vi "NI 5783 - Getting Started (FPGA).vi"() -> ()   [LabVIEW 2017]
doc: "Example Description:\nThis example acquires records of analog input data and generates analog output data from the NI 5783 adapter module. For the analog input, it allows the user to select an AI channel, trigger type, and record size. For the analog output, it allows the user to select AO channel, waveform signal type, frequency, amplitude, and sampling information. This VI is compiled for all FPGA targets by default.\n\nRunning the VI:\nThis VI must be run from the NI 5783 - Getting Started (Host).vi. Refer to the host VI documentation for steps regarding running and configuring the FPGA VI. \n\nExecution Steps:\nRefer to the Block Diagram of this VI for execution comments."
uses:
  Program Files (x86)/National Instruments/LabVIEW 2017/examples/FlexRIO/IO Modules/NI 5783/NI 5783 - Getting Started/Controls/AI Trigger Type.ctl
  <instrlib>/_niInstr/Streaming/v1/Common/Stream State.ctl
  <instrlib>/_niInstr/Data Trigger/v1/Shared/Public/Level Configuration I16.ctl
  <instrlib>/_niInstr/Data Trigger/v1/Shared/Public/Level Configuration Trigger When.ctl
  <vilib>/Platform/TimedLoop/XDataNode/timing_clust.ctl
  <vilib>/Platform/TimedLoop/XDataNode/nitl_modes.ctl
  <vilib>/Platform/TimedLoop/XDataNode/wakeup.ctl
  <vilib>/rvi/Emulation/niFpgaSctlEmulationGetInTimedLoop.vi
  <vilib>/rvi/Emulation/niFpgaEmulationReportErrorSimple.vi
  <vilib>/rvi/Emulation/niFpgaGetClockAttributes.vi
  <vilib>/rvi/Emulation/niFpgaCriticalErrorInLSC.vi
  <vilib>/rvi/eio/common/nirviEmuTemplateMethod_errors.vi
  <instrlib>/_niInstr/Data Trigger/v1/FPGA/Private/Trigger/Level I16xNspc.vi
  <vilib>/rvi/interface/RandomDataEmulation/nirviRandomDataMultiElementFPGAFIFO.vi
  <instcachedir>/0/nirviRandomDataMultiElementFPGAFIFO_6740B454F3C245F78F76ED91F73FD8DB.lvgen/nirviRandomDataMultiElementFPGAFIFO_6740B454F3C245F78F76ED91F73FD8DB_000.vi
  <vilib>/rvi/interface/RandomDataEmulation/niFpgaRandomDataHandleErrors.vi
  <vilib>/Platform/TimedLoop/XDataNode/XDataNode.xnode
  <vilib>/eio/EIONode/EIONode.xnode
  <vilib>/rvi/DataTransferAndStorage/Container/XNode/niFpgaContainer.xnode
  <vilib>/rvi/interface/RandomDataEmulation/nirviRandomDataFpgaMultiElementTemplate.vi
  <vilib>/Platform/TimedLoop/XDataNode/XDNodeRunTimeDep.lvlib
  <instrlib>/_niInstr/Streaming/v1/FPGA/niInstr Streaming v1 FPGA.lvlib
  <instrlib>/_niInstr/Basic Elements/v1/FPGA/niInstr Basic Elements v1 FPGA.lvlib
  <instrlib>/_niInstr/Data Trigger/v1/FPGA/niInstr Data Trigger v1 FPGA.lvlib
  <instrlib>/_niInstr/Streaming/v1/Common/niInstr Streaming v1 Common.lvlib
  <instrlib>/_niInstr/Data Trigger/v1/Shared/niInstr Data Trigger v1 Shared.lvlib
panel:
  in  "Trigger Configuration":T1
  out "IO Module\\User Command Return Valid":bool
  out "IO Module\\User Command Return":u32
  out "IO Module\\User Command Error":u16
  in  "IO Module\\User Command Arg 1":u32
  in  "IO Module\\User Command Arg 0":u32
  out "IO Module\\User Command Ready":bool
  in  "IO Module\\User Command Valid":bool
  in  "IO Module\\User Command":u32
  out "IO Module\\User Error":u32
  in  "stream.num samples 0":u64
  out "stream.state 0":T3
  out "stream.samples transferred 0":u64
  in  "stream.request state 0":T3
  out "stream.metadata 0":u64
  in  "Trigger Type":T4
  out "IO Module\\InitDone":bool
  # "Refer to the Block Diagram of this VI for execution comments."
  # "For other instructions, select Help>>Show Context Help and move the cursor over the VI icon to display help for this VI."
  # "Analog Input"
  # "Analog Output"
  # "Resource Configuration"
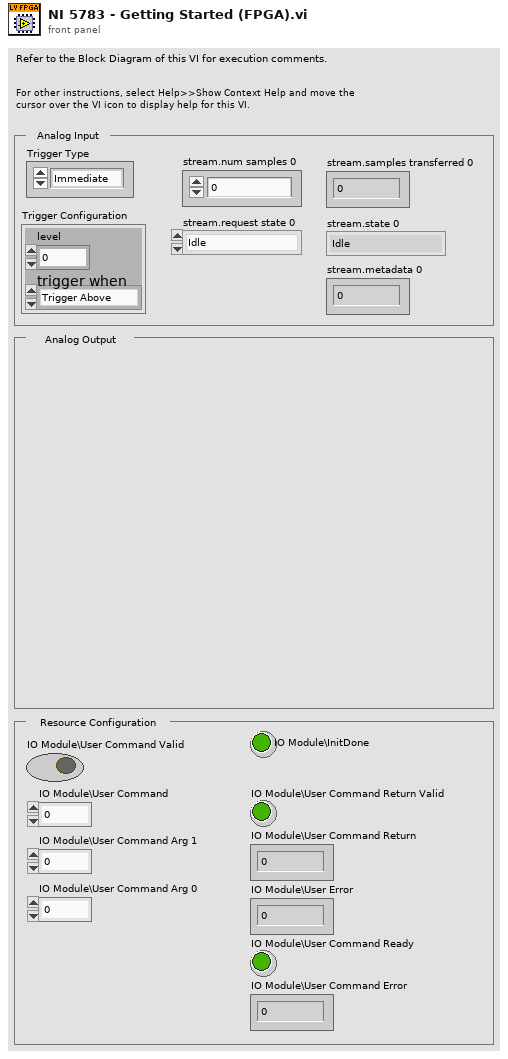
[diagram p1: front panel]
types:
  T1 = typedef "niInstr Data Trigger v1 Shared.lvlib/Level Configuration I16.ctl" = cluster{"level":i16, "trigger when":T2}
  T2 = typedef "niInstr Data Trigger v1 Shared.lvlib/Level Configuration Trigger When.ctl" = enum8{"Trigger Above", "Trigger Below"}
  T3 = typedef "niInstr Streaming v1 Common.lvlib/Stream State.ctl" = enum8{"Idle", "Finite Transfer", "Continuous", "Done", "Error", "Not Ready", "Cancel"}
  T4 = typedef "AI Trigger Type.ctl" = enum8{"Immediate", "Data Trigger", "TRIG input"}
  T5 = typedef "XDNodeRunTimeDep.lvlib/timing_clust.ctl" = cluster{"Expected End [f-1]":u64, "Actual End [f-1]":u64, "Finished Late? [f-1]":bool, "Expected End [i-1]":u64, "Actual End [i-1]":u64, "Finished Late? [i-1]":bool, "Expected Start [i]":u64, "Actual Start [i]":u64, "Expected Start [f]":u64, "Actual Start [f]":u64, "Source Name":string, "Structure Name":string, "Period":i64, "Deadline":i64, "Offset":i64, "Start":i64, "Priority":i32, "Timeout":i32, "Mode":T6, "Wakeup Reason":T7, "Error":errorcluster, "Source Type":string, "Secondary Source Type":string, "Global End Time":u64, "Global Start Time":u64, "Frame Duration":u64, "Iteration Duration":u64, "Assigned CPU":i32, "I/O Scan Engine Mode":u32}
  T6 = typedef "XDNodeRunTimeDep.lvlib/nitl_modes.ctl" = enum32{"No Change", "Process missed periods, maintain original phase", "Discard missed periods, maintain original phase", "Process missed periods, ignore original phase", "Discard missed periods, ignore original phase"}
  T7 = typedef "XDNodeRunTimeDep.lvlib/wakeup.ctl" = enum32{"Normal", "Aborted", "Asynchronous wakeup", "Timing source error", "Timed loop error", "Timeout"}
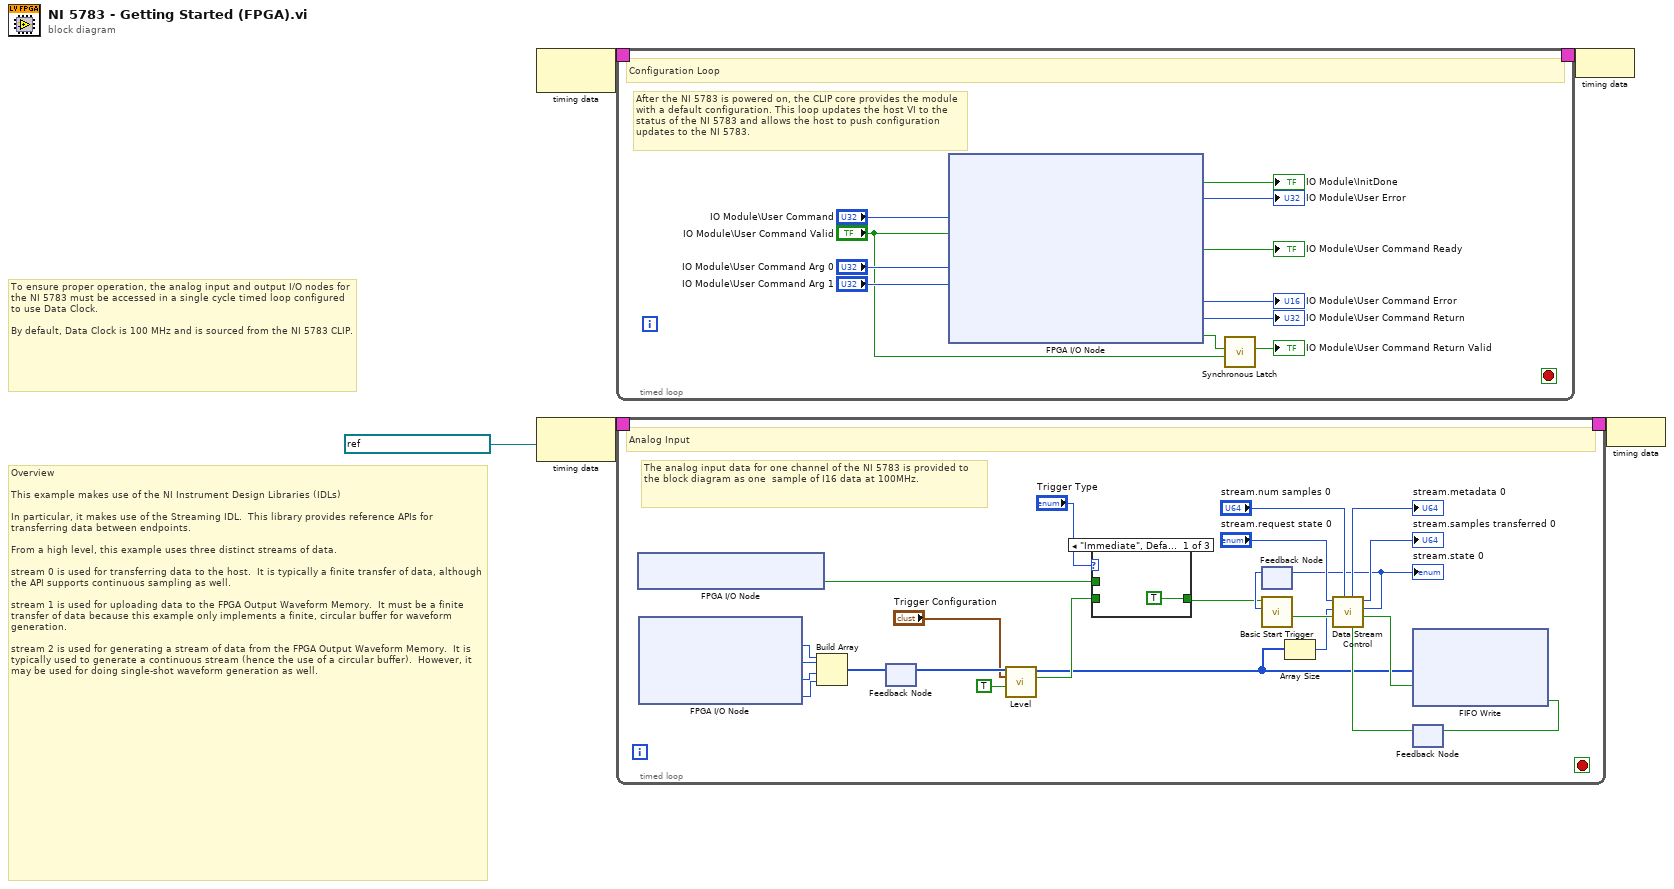
[diagram p0: block diagram]
diagram:
  # "Overview\n\nThis example makes use of the NI Instrument Design Libraries (IDLs)\n\nIn particular, it makes use of the Streaming IDL.  This library provides reference APIs for transferring data between endpoints.\n\nFrom a high level, this example uses three distinct streams of data.\n\nstream 0 is used for transferring data to the host.  It is typically a finite transfer of data, although the API supports continuous sampling as well.\n\nstream 1 is used for uploading data to the FPGA Output Waveform Memory.  It must be a finite transfer of data because this example only implements a finite, circular buffer for waveform generation.\n\nstream 2 is used for generating a stream of data from the FPGA Output Waveform Memory.  It is typically used to generate a continuous stream (hence the use of a circular buffer).  However, it may be used for doing single-shot waveform generation as well."
  # "To ensure proper operation, the analog input and output I/O nodes for the NI 5783 must be accessed in a single cycle timed loop configured to use Data Clock. \n\nBy default, Data Clock is 100 MHz and is sourced from the NI 5783 CLIP."
  n1 = node-c288() -> (w2:T5)  [unwired: 1 in]
  n2 = node-c288(refnum<k21> "IO Module\\Data Clock" ("Source Name")) -> (w5:T5)
  n3 = timed-loop {
    timing: w2 -> [_]
    timing-out: [_] -> w1
    stop <- _ stop-if-true
    # "After the NI 5783 is powered on, the CLIP core provides the module with a default configuration. This loop updates the host VI to the status of the NI 5783 and allows the host to push configuration updates to the NI 5783."
    # "Configuration Loop"
    n4 = xnode "FPGA I/O Node"("IO Module\\User Command"="IO Module\\User Command", "IO Module\\User Command Valid"="IO Module\\User Command Valid", "IO Module\\User Command Arg 0"="IO Module\\User Command Arg 0", "IO Module\\User Command Arg 1"="IO Module\\User Command Arg 1") -> ("IO Module\\InitDone"=→"IO Module\\InitDone":bool, "IO Module\\Clip Error Code"=→"IO Module\\User Error":u32, "IO Module\\User Command Ready"=→"IO Module\\User Command Ready":bool, "IO Module\\User Command Error"=→"IO Module\\User Command Error":u16, "IO Module\\User Command Return"=→"IO Module\\User Command Return":u32, "IO Module\\User Command Return Valid"=w7:bool)  [unwired: 10 in, 10 out]
    n5 = call <instrlib>:"Synchronous Latch.vi"("clear"="IO Module\\User Command Valid", "set"=w7) -> ("out"=→"IO Module\\User Command Return Valid":bool)  [unwired: 9 in]
  }
  n6 = timed-loop {
    timing: w5 -> [_]
    timing-out: [_] -> w4
    stop <- _ stop-if-true
    # "The analog input data for one channel of the NI 5783 is provided to the block diagram as one  sample of I16 data at 100MHz."
    # "Analog Input"
    n7 = xnode "FPGA I/O Node"() -> ("IO Module\\Trigger Rd Data"=w25:bool)  [unwired: 1 in, 1 out]
    n8 = xnode "FPGA I/O Node"() -> ("IO Module\\AI 0 Data N"=w30:i16, "IO Module\\AI 1 Data N"=w29:i16, "IO Module\\AI 2 Data N"=w28:i16, "IO Module\\AI 3 Data N"=w27:i16)  [unwired: 4 in, 4 out]
    n9 = Build Array(w30, w29, w28, w27) -> (w26:i16[])
    n10 = feedback-in #1(w26) -> ()
    n11 = feedback #1() -> (w24:i16[])  [unwired: 1 in]
    n12 = call-poly <instrlib>:"Level.vi"("data in"=w24, "configuration"="Trigger Configuration", "input valid"=TRUE) -> ("data out"=w19:i16[], "trigger"=w23:bool)  [unwired: 7 in, 4 out]
    n13 = case shown="\"Immediate\", Default" "Trigger Type" {
      tunnel: w23 -> [_ w44 _]
      tunnel: [TRUE ("Trigger") w44 w45] -> w31
      tunnel: w25 -> [_ _ w45]
      frame "Immediate", Default {
      }
      frame "Data Trigger" {
      }
      frame "TRIG input" {
      }
    }
    n14 = feedback #2() -> (w37:T3)  [unwired: 1 in]
    n15 = call <instrlib>:"Basic Start Trigger.vi"("stream.state"=w37, "start trigger"=w31) -> ("data valid"=w38:bool)  [unwired: 9 in]
    n16 = Array Size(array=w19) -> (size(s)=w20:i32)
    n17 = feedback #3() -> (w33:bool)  [unwired: 1 in]
    n18 = call <instrlib>:"Data Stream Control.vi"("ready for input?"=w33, "stream.num samples 0"="stream.num samples 0", "data valid"=w38, "element count"=w20, "stream.request state 0"="stream.request state 0") -> ("send data"=w35:bool, "stream.state 0"=w36:T3, "stream.samples transferred 0"=→"stream.samples transferred 0":u64, "stream.metadata 0"=→"stream.metadata 0":u64)  [unwired: 2 in, 1 out]
    "stream.state 0" <- w36
    n19 = feedback-in #2(w36) -> ()
    n20 = xnode ("FIFO Write")("Element"=w19, "Input Valid"=w35) -> ("Ready for Input"=w34:bool)  [unwired: 1 in, 1 out]
    n21 = feedback-in #3(w34) -> ()
  }
  n22 = node-c288(w1) -> ()
  n23 = node-c288(w4) -> ()
